vi "CheckIfGObjectMatches.vi"(8 "error in (no error)":errorcluster, 10 "GObj Refnum":refnum<vi>, 11 "Decoration Layout in":refnum<class "Decoration Layout.lvclass">) -> (0 "error out":errorcluster, 2 "compatible?":bool)   [LabVIEW 2010, in "NI_SE_Front Panel Layout.lvlib" / "Decoration Layout.lvclass"]
uses:
  Decoration Layout.lvclass
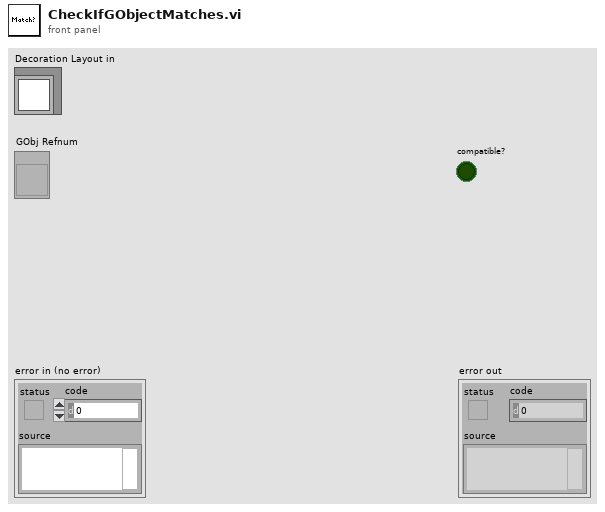
[diagram p1: front panel]
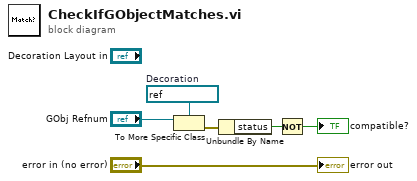
[diagram p0: block diagram]
diagram:
  w5 = refnum<vi> refnum  # Decoration
  n1 = To More Specific Class(target class=w5, reference="GObj Refnum") -> (error out=w4:errorcluster)  [unwired: 1 in, 1 out]
  n2 = Unbundle By Name(w4) -> ("status"=w3:bool)
  n3 = Not(x=w3) -> (.not. x?=→"compatible?":bool)
  "error out" <- "error in (no error)"
